vi "LINE_v2.vi"() -> ()   [LabVIEW 2010]
uses:
  <vilib>/express/express arith-compare/Formula/XNode/ExpressFormulaBlockNode.xnode
panel:
  in  "x-dist":i32
  in  "Motor GPIB":u8=6
  in  "speed":u16
  in  "y-dist":i32
  in  "Current (mA)":dbl
  in  "Laser GPIB":u8=10 max=100
  out "Dummy":string
  # "LINE<space>[Displacement]<space>[Speed]<space>[Current]"
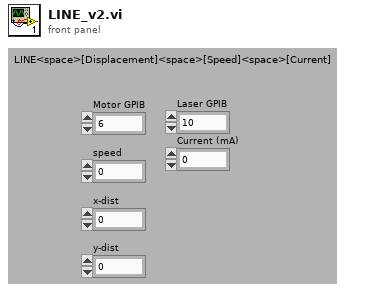
[diagram p1: front panel]
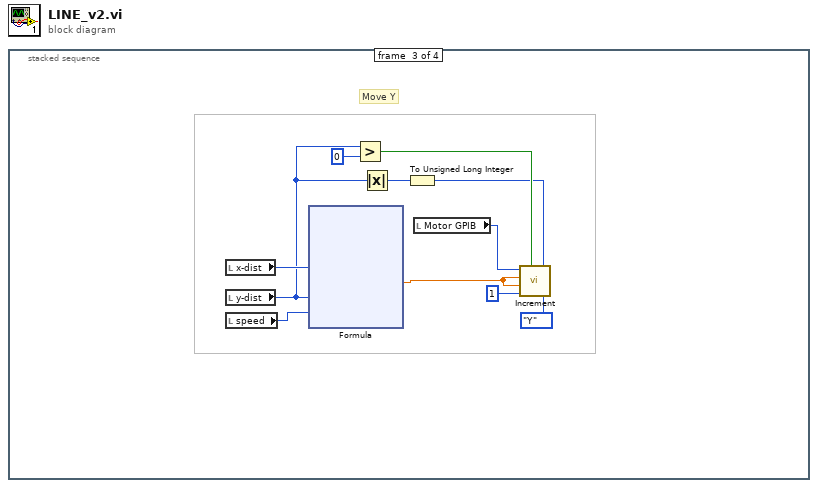
[diagram p0: block diagram]
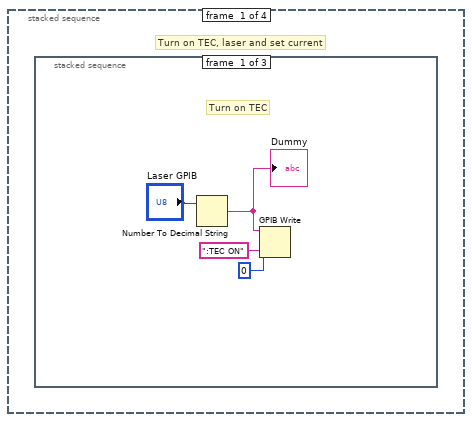
[diagram p2: hidden frame]
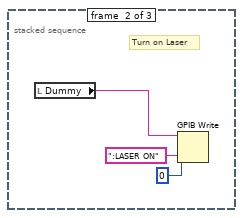
[diagram p3: hidden frame]
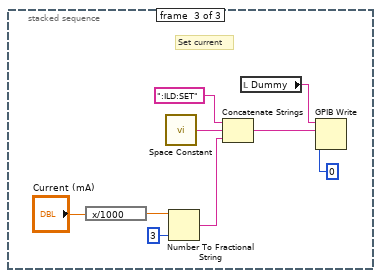
[diagram p4: hidden frame]
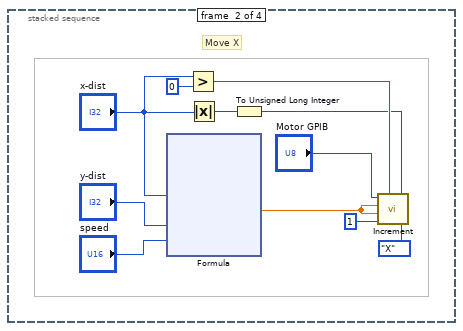
[diagram p5: hidden frame]
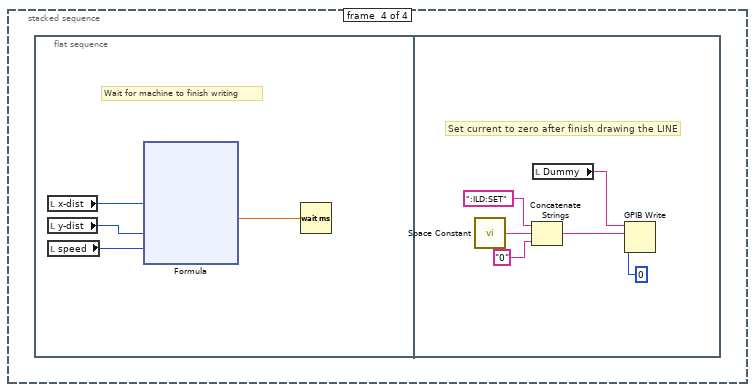
[diagram p6: hidden frame]
diagram:
  n1 = stacked-sequence {
    frame #0 {
      # "Turn on TEC, laser and set current"
      n2 = stacked-sequence {
        frame #0 {
          # "Turn on TEC"
          n3 = Number To Decimal String(number="Laser GPIB") -> (decimal integer string=w1:string)  [unwired: 1 in]
          "Dummy" <- w1
          n4 = GPIB Write(0:w1, 1:":TEC ON" ("data"), 2:i16 0 ("mode (0)")) -> ()  [unwired: 2 in, 2 out]
        }
        frame #1 {
          # "Turn on Laser"
          n5 = local read "Dummy"() -> (w5:string)
          n6 = GPIB Write(0:w5, 1:":LASER ON" ("data"), 2:i16 0 ("mode (0)")) -> ()  [unwired: 2 in, 2 out]
        }
        frame #2 {
          # "Set current"
          n7 = expression code="x/1000"("Current (mA)") -> (w12:dbl)
          n8 = call <vilib>:"Space Constant.vi"() -> ("String"=w14:string)
          n9 = Number To Fractional String(number=w12, precision (6)=i16 3) -> (F-format string=w9:string)  [unwired: 2 in]
          n10 = Concatenate Strings(":ILD:SET", w14, w9) -> (w13:string)
          n11 = local read "Dummy"() -> (w8:string)
          n12 = GPIB Write(0:w8, 1:w13, 2:i16 0 ("mode (0)")) -> ()  [unwired: 2 in, 2 out]
        }
      }
    }
    frame #1 {
      # "Move X"
      n13 = xnode "Formula"("X1"="x-dist", "X2"="y-dist", "X3"="speed") -> ("Result"=w23:dbl)  [unwired: 1 in, 1 out]
      n14 = Greater?(x="x-dist", y=0) -> (0:w21:bool)
      n15 = Absolute Value(x="x-dist") -> (abs(x)=w18:i32)
      n16 = To Unsigned Long Integer(number=w18) -> (unsigned 32bit integer=w17:u32)
      n17 = call "Increment.vi"("GPIB_Addr"="Motor GPIB", "F Speed"=w23, "L Speed"=w23, "Rate"=u16 1, "CCW 3"=w21, "Distance"=w17, "Axis"=enum16{"X", "Y", "Z", "U", "V", "W"}."X") -> ()
    }
    frame #2 {
      # "Move Y"
      n18 = local read "x-dist"() -> (w44:i32)
      n19 = local read "y-dist"() -> (w41:i32)
      n20 = local read "speed"() -> (w48:u16)
      n21 = xnode "Formula"("X1"=w44, "X2"=w41, "X3"=w48) -> ("Result"=w43:dbl)  [unwired: 1 in, 1 out]
      n22 = Greater?(x=w41, y=0) -> (0:w45:bool)
      n23 = Absolute Value(x=w41) -> (abs(x)=w42:i32)
      n24 = To Unsigned Long Integer(number=w42) -> (unsigned 32bit integer=w40:u32)
      n25 = local read "Motor GPIB"() -> (w47:u8)
      n26 = call "Increment.vi"("GPIB_Addr"=w47, "F Speed"=w43, "L Speed"=w43, "Rate"=u16 1, "CCW 3"=w45, "Distance"=w40, "Axis"=enum16{"X", "Y", "Z", "U", "V", "W"}."Y") -> ()
    }
    frame #3 {
      n27 = flat-sequence {
        frame #0 {
          # "Wait for machine to finish writing"
          n28 = local read "x-dist"() -> (w66:i32)
          n29 = local read "y-dist"() -> (w65:i32)
          n30 = local read "speed"() -> (w64:u16)
          n31 = xnode "Formula"("X1"=w66, "X2"=w65, "X3"=w64) -> ("Result"=w63:dbl)  [unwired: 1 in, 1 out]
          n32 = Wait (ms)(milliseconds to wait=w63) -> ()  [unwired: 1 out]
        }
        frame #1 {
          # "Set current to zero after finish drawing the LINE"
          n33 = call <vilib>:"Space Constant.vi"() -> ("String"=w82:string)
          n34 = Concatenate Strings(":ILD:SET", w82, "0" ("string")) -> (w81:string)
          n35 = local read "Dummy"() -> (w79:string)
          n36 = GPIB Write(0:w79, 1:w81, 2:i16 0 ("mode (0)")) -> ()  [unwired: 2 in, 2 out]
        }
      }
    }
  }
